vi "Instrument Type ID.vi"() -> (1 "instrument type id":string)   [LabVIEW 2021, in "Session Management niSwitch.lvlib"]
uses:
  Session Management niSwitch.lvlib
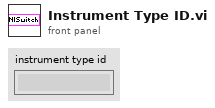
[diagram p1: front panel]
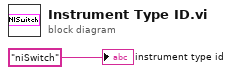
[diagram p0: block diagram]
diagram:
  "instrument type id" <- "niSwitch" ("instrument type id")
